vi "Find first empty row.vi"(8 "error in (no error)":errorcluster, 11 "Excel Sheet in":refnum<class "Excel Sheet.lvclass">) -> (0 "error out":errorcluster, 2 "Next Empty Row":i32, 3 "Excel Sheet out":refnum<class "Excel Sheet.lvclass">)   [LabVIEW 2016, in "Excel Sheet.lvclass"]
uses:
  Excel Sheet.lvclass
  Excel Sheet.lvclass/Excel Sheet.ctl
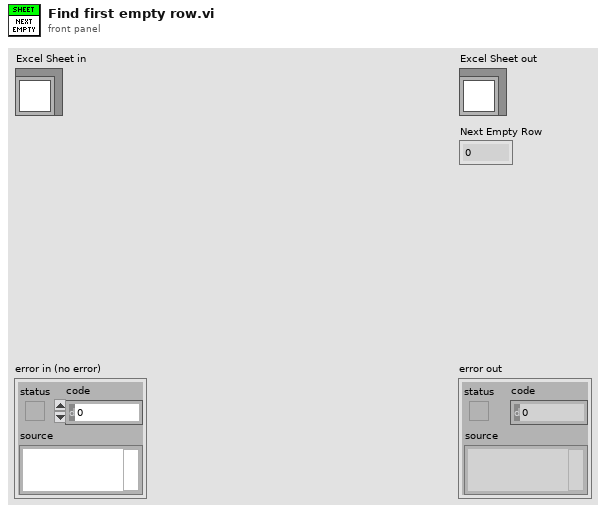
[diagram p1: front panel]
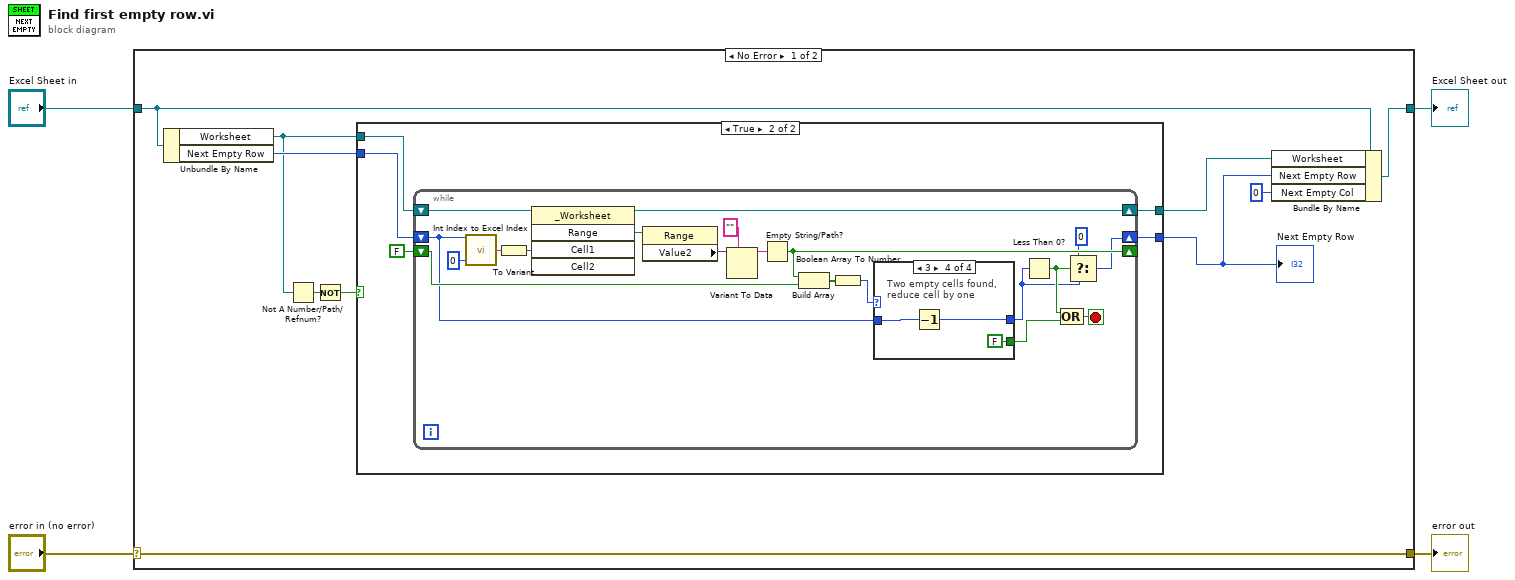
[diagram p0: block diagram]
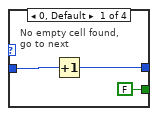
[diagram p3: hidden frame]
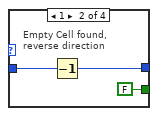
[diagram p4: hidden frame]
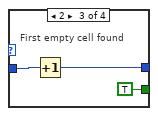
[diagram p5: hidden frame]
diagram:
  n1 = case shown="No Error" "error in (no error)" {
    selector: "error in (no error)" -> [w14 w55]
    tunnel: [w14 w55] -> w3
    tunnel: [w11 w54] -> w1
    tunnel: "Excel Sheet in" -> [w12 w54]
    frame No Error {
      n2 = Unbundle By Name(w12) -> ("Worksheet"=w9:refnum<k7>, "Next Empty Row"=w13:i32)
      n3 = Not A Number/Path/Refnum?(number/path/refnum=w9) -> (NaN/Path/Refnum?=w8:bool)
      n4 = Not(x=w8) -> (.not. x?=w7:bool)
      n5 = case shown="True" w7 {
        tunnel: w9 -> [w16 w21]
        tunnel: w13 -> [w15 w19]
        tunnel: [w15 w18] -> w5
        tunnel: [w16 w17] -> w10
        frame False {
        }
        frame True {
          n6 = while {
            shift-right: [w25] -> w18
            shift-left: w19 -> [w30]
            shift-right: [w34] -> _
            shift-left: FALSE -> [w33]
            shift-right: [w22] -> w17
            shift-left: w21 -> [w27]
            stop <- w28 stop-if-true
            n7 = call "Int Index to Excel Index.vi"("Column"=0, "Row"=w30) -> ("Cell"=w40:string)  [unwired: 3 in]
            n8 = To Variant(anything=w40) -> (Variant=w39:variant)
            n9 = invoke class="_Worksheet" method="Range"(reference=w27, "Cell1"=w39) -> (reference out=w22:refnum<k7>, "Range"=w38:refnum<k7>)  [unwired: 3 in, 3 out]
            n10 = property class="Range"(reference=w38) -> ("Value2"=w35:variant)  [unwired: 1 in, 2 out]
            n11 = Variant To Data(type="", Variant=w35) -> (data=w37:string)  [unwired: 1 in, 1 out]
            n12 = Empty String/Path?(string/path=w37) -> (empty?=w34:bool)
            n13 = Build Array(w34, w33) -> (w32:bool[])
            n14 = Boolean Array To Number(Boolean array=w32) -> (number=w31:u32)
            n15 = case shown="3" w31 {
              tunnel: w30 -> [w44 w47 w50 w53]
              tunnel: [w43 w46 w49 w52] -> w24
              tunnel: [FALSE FALSE TRUE FALSE] -> w29
              frame 0, Default {
                # "No empty cell found, \ngo to next"
                n16 = Increment(x=w44) -> (x+1=w43:i32)
              }
              frame 1 {
                # "Empty Cell found,\nreverse direction"
                n17 = Decrement(x=w47) -> (x-1=w46:i32)
              }
              frame 2 {
                # "First empty cell found"
                n18 = Increment(x=w50) -> (x+1=w49:i32)
              }
              frame 3 {
                # "Two empty cells found,\nreduce cell by one"
                n19 = Decrement(x=w53) -> (x-1=w52:i32)
              }
            }
            n20 = Less Than 0?(x=w24) -> (x < 0?=w26:bool)
            n21 = Compound Arithmetic op=OR(w26, w29) -> (w28:bool)
            n22 = Select(t=0, s=w26, f=w24) -> (s? t:f=w25:i32)
          }
        }
      }
      "Next Empty Row" <- w5
      n23 = Bundle By Name(cluster=w12, "Worksheet"=w10, "Next Empty Row"=w5, "Next Empty Col"=0) -> (w11:refnum<class "Excel Sheet.lvclass">)
    }
    frame Error {
    }
  }
  "error out" <- w3
  "Excel Sheet out" <- w1
